vi "Initialize_Image_with_Random_Name-3.vi"(2 "error IN":errorcluster, 3 "Image Type":T2 items=["Grayscale (U8)", "Grayscale (I16)", "Grayscale (SGL)", "Complex (CSG)", "RGB (U32)", "HSL (U32)", "RGB (U64)", "Grayscale (U16)"], 4 "Unique ID":string) -> (0 "error OUT":errorcluster, 1 "[OUT] New Image":T1)   [LabVIEW 2017]
uses:
  <vilib>/vision/Image Controls.llb/IMAQ Image.ctl
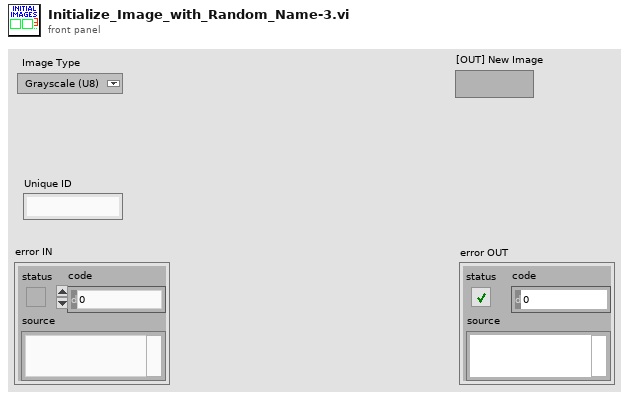
[diagram p1: front panel]
types:
  T1 = typedef "IMAQ Image.ctl" = refnum<image>
  T2 = typedef "Image Type" = u32
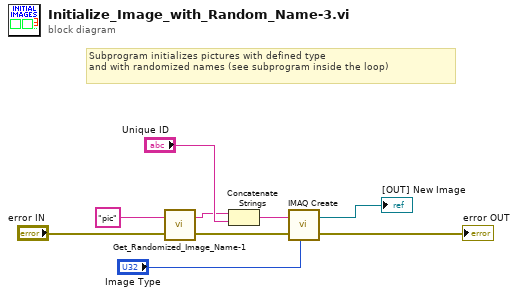
[diagram p0: block diagram]
diagram:
  # "Subprogram initializes pictures with defined type \nand with randomized names (see subprogram inside the loop)"
  n1 = call "Get_Randomized_Image_Name-1.vi"("error IN"="error IN", "Main Name"="pic") -> ("error OUT"=w4:errorcluster, "Randomized name"=w2:string)
  n2 = Concatenate Strings(w2, "Unique ID") -> (w3:string)
  n3 = call "IMAQ Create"("Image Name"=w3, "Image Type"="Image Type", "error in (no error)"=w4) -> ("New Image"=→"[OUT] New Image":T1, "error out"=→"error OUT":errorcluster)  [unwired: 2 in]
